vi "Write tcp connection.vi"(8 "error in (no error)":errorcluster, 10 "tcp connection":refnum<k5>, 11 "TCP Interface in":refnum<class "TCP Interface.lvclass">) -> (0 "error out":errorcluster, 3 "TCP Interface out":refnum<class "TCP Interface.lvclass">)   [LabVIEW 2021, in "TCP Interface.lvclass"]
uses:
  TCP Interface.lvclass
  TCP Interface.lvclass/TCP Interface.ctl
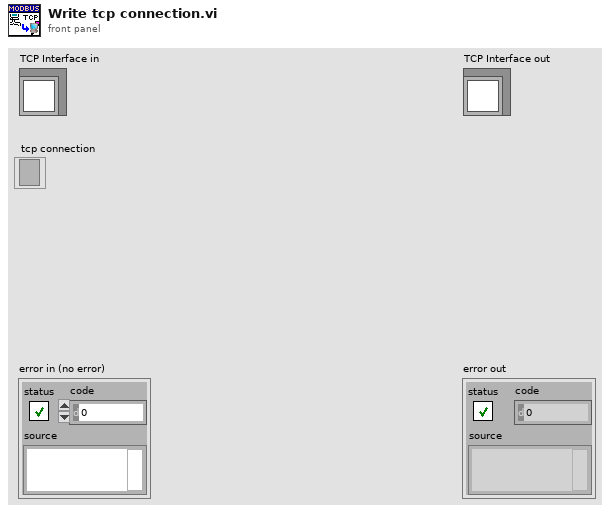
[diagram p1: front panel]
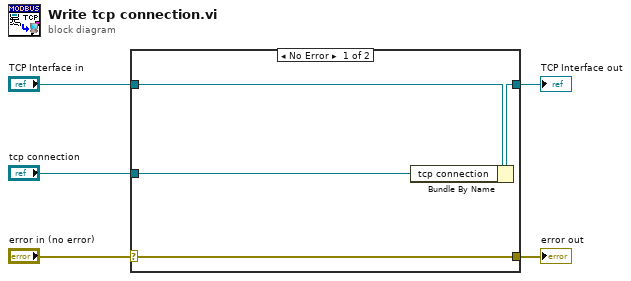
[diagram p0: block diagram]
diagram:
  n1 = case shown="No Error" "error in (no error)" {
    selector: "error in (no error)" -> [w9 w10]
    tunnel: [w9 w10] -> w4
    tunnel: [w7 w11] -> w2
    tunnel: "TCP Interface in" -> [w8 w11]
    tunnel: "tcp connection" -> [w6 _]
    frame No Error {
      n2 = Bundle By Name(cluster=w8, "tcp connection"=w6) -> (w7:refnum<class "TCP Interface.lvclass">)
    }
    frame Error {
    }
  }
  "error out" <- w4
  "TCP Interface out" <- w2
